vi "getLogicInChannel.vi"(8 "error in (no error)":errorcluster, 11 "pHandle":u32) -> (0 "error out":errorcluster, 1 "return type":i32, 2 "sensitivtyStr":string, 3 "inputTypeStr":string)   [LabVIEW 2011, in "sbgLabView.lvlib"]
uses:
  sbgLabView.lvlib
  sbgMatLab.dll
panel:
  out "nsDelay":i32
  out "locationStr":string
  in  "channel":u8
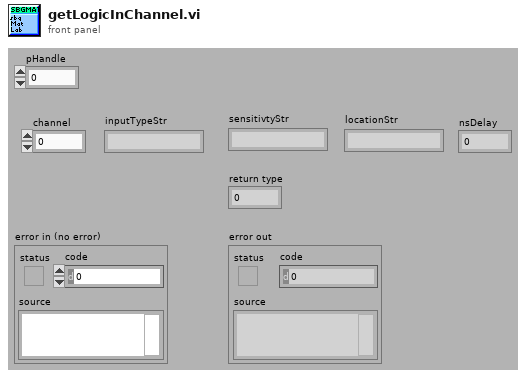
[diagram p1: front panel]
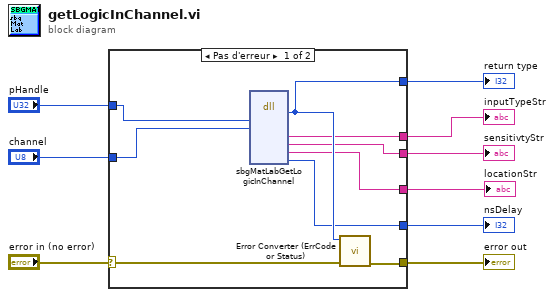
[diagram p0: block diagram]
diagram:
  n1 = case shown="Pas d'erreur" "error in (no error)" {
    selector: "error in (no error)" -> [w14 w19]
    tunnel: [w13 w19] -> w8
    tunnel: [w18 _] -> w7
    tunnel: "pHandle" -> [w17 _]
    tunnel: [w16 _] -> w5
    tunnel: [w15 _] -> w4
    tunnel: [w12 _] -> w3
    tunnel: "channel" -> [w11 _]
    tunnel: [w10 _] -> w1
    frame No Error {
      n2 = dll-call lib="C:/SBG-Systems/remote/projects/software/projects/labviewExample/sbgLabView/sbgMatLab.*" fn="sbgMatLabGetLogicInChannel" ("sbgMatLab.dll:sbgMatLabGetGpsOptions")("pHandle"=w17, "channel"=w11) -> ("type de retour"=w18:i32, "inputTypeStr"=w16:string, "sensitivityStr"=w15:string, "locationStr"=w10:string, "pNsDelay"=w12:i32)  [unwired: 9 in, 2 out]
      n3 = call "Error Converter (ErrCode or Status).vi"("error in (no error)"=w14, "error code"=w18) -> ("error out"=w13:errorcluster)  [unwired: 9 in]
    }
    frame Error {
    }
  }
  "return type" <- w7
  "inputTypeStr" <- w5
  "sensitivtyStr" <- w4
  "error out" <- w8
  "locationStr" <- w1
  "nsDelay" <- w3
